vi "Read Data.vi"(8 "error in (no error)":errorcluster, 11 "Boolean Data in":refnum<class "Boolean Data.lvclass">) -> (0 "error out":errorcluster, 2 "Data":bool, 3 "Boolean Data out":refnum<class "Boolean Data.lvclass">)   [LabVIEW 2013, in "Boolean Data.lvclass"]
uses:
  Boolean Data.lvclass
  Boolean Data.lvclass/Boolean Data.ctl
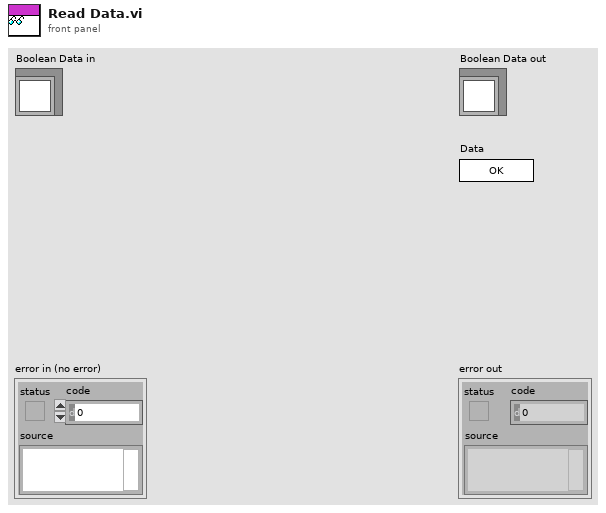
[diagram p1: front panel]
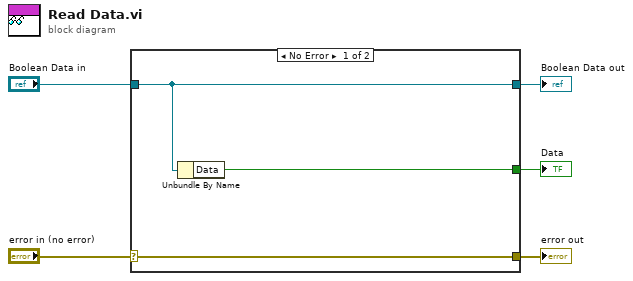
[diagram p0: block diagram]
diagram:
  n1 = case shown="No Error" "error in (no error)" {
    selector: "error in (no error)" -> [w8 w9]
    tunnel: [w8 w9] -> w4
    tunnel: [w7 w10] -> w2
    tunnel: "Boolean Data in" -> [w7 w10]
    tunnel: [w6 _] -> w1
    frame No Error {
      n2 = Unbundle By Name(w7) -> ("Data"=w6:bool)
    }
    frame Error {
    }
  }
  "error out" <- w4
  "Boolean Data out" <- w2
  "Data" <- w1
